vi "Configure Bus Source (Parallel).vi"(0 "VISA resource name":refnum<visa-resource-name>, 1 "Parallel Width (20)":dbl=20.0, 2 "Lock Clock":bool, 5 "BUS Number (9: Bus 1)":u16(ring)=9 items=["Bus 1"=9, "Bus 2"=10, "Bus 3"=11, "Bus 4"=12], 7 "Bit Source (0: Channel 1)":u16(ring) items=["Channel 1"=0, "Channel 2"=1, "Channel 3"=2, "Channel 4"=3, "Digital Channel 0"=14, "Digital Channel 1"=15, "Digital Channel 2"=16, "Digital Channel 3"=17, "Digital Channel 4"=18, "Digital Channel 5"=19, "Digital Channel 6"=20, "Digital Channel 7"=21, "Digital Channel 8"=22, "Digital Channel 9"=23, "Digital Channel 10"=24, "Digital Channel 11"=25, "Digital Channel 12"=26, "Digital Channel 13"=27, "Digital Channel 14"=28, "Digital Channel 15"=29], 9 "Clock Source (0: Channel 1)":u16(ring) items=["Channel 1"=0, "Channel 2"=1, "Channel 3"=2, "Channel 4"=3, "Digital Channel 0"=14, "Digital Channel 1"=15, "Digital Channel 2"=16, "Digital Channel 3"=17, "Digital Channel 4"=18, "Digital Channel 5"=19, "Digital Channel 6"=20, "Digital Channel 7"=21, "Digital Channel 8"=22, "Digital Channel 9"=23, "Digital Channel 10"=24, "Digital Channel 11"=25, "Digital Channel 12"=26, "Digital Channel 13"=27, "Digital Channel 14"=28, "Digital Channel 15"=29], 11 "error in (no error)":errorcluster, 12 "Bit Number (0: Normal)":u16(ring) items=["0", "1", "2", "3", "4", "5", "6", "7"], 13 "Clock Edge (0: Either)":u16(ring) items=["Either", "Rising", "Falling"]) -> (4 "VISA resource name out":refnum<visa-resource-name>, 15 "error out":errorcluster)   [LabVIEW 2010, in "Tektronix DPO MSO 2000 4000 Series.lvlib"]
doc: "This VI configures the Parallel bus.\n\n<B>Note:</B> This VI is only applicable for MSO3000 series."
uses:
  <instrlib>/Tektronix DPO MSO 2000 4000 Series/Tektronix DPO MSO 2000 4000 Series.lvlib
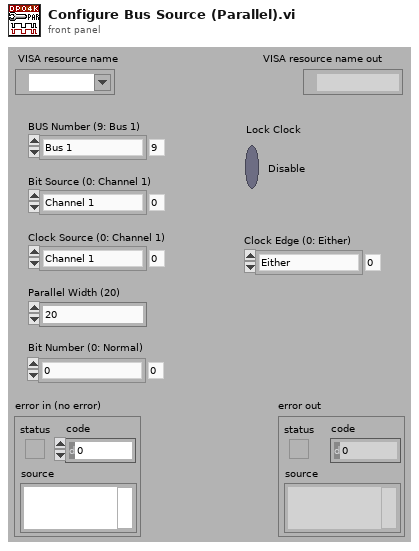
[diagram p1: front panel]
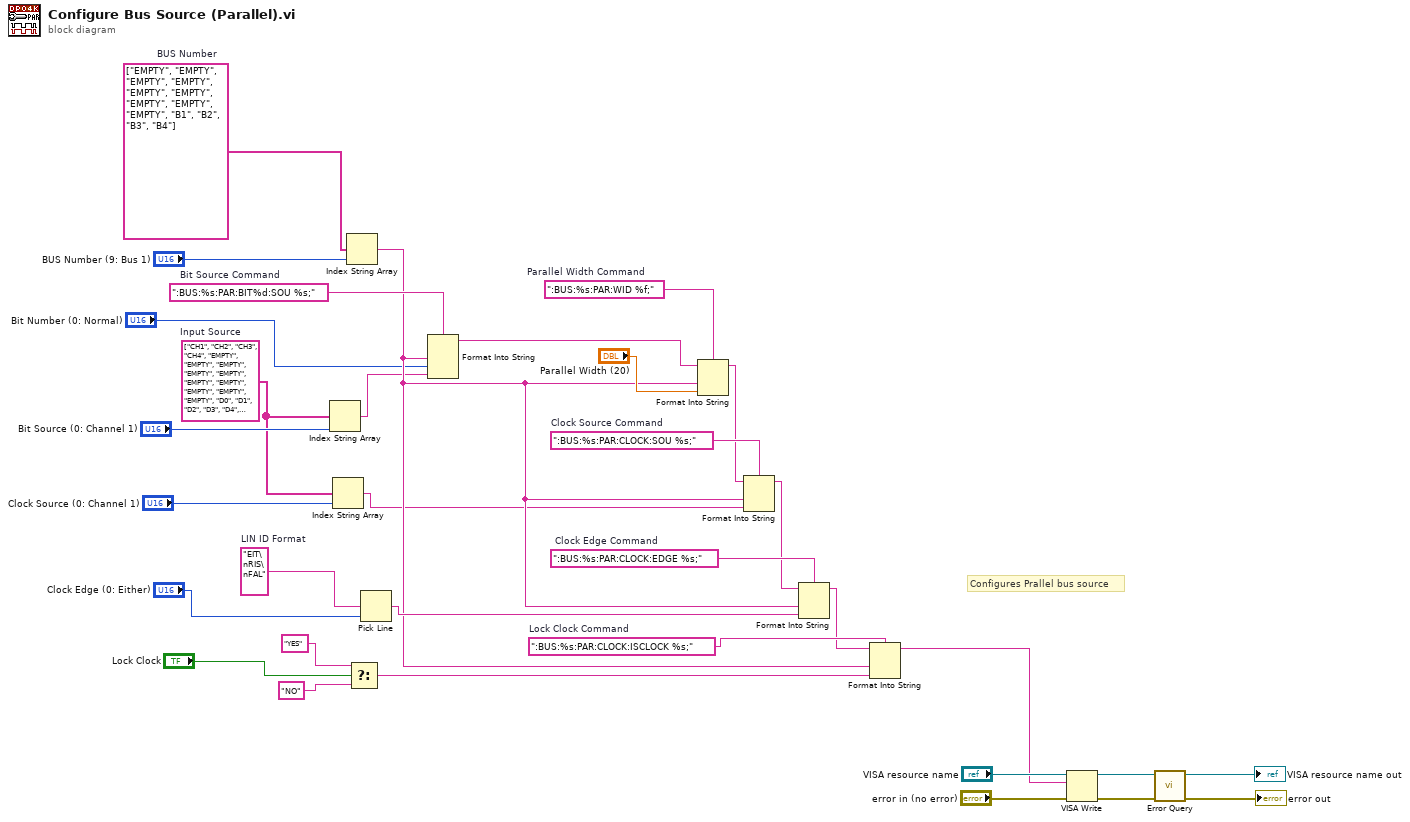
[diagram p0: block diagram]
diagram:
  w8 = string[] ["CH1", "CH2", "CH3", "CH4", "EMPTY", "EMPTY", "EMPTY", "EMPTY", "EMPTY", "EMPTY", "EMPTY", "EMPTY", "EMPTY", "EMPTY", "D0", "D1", "D2", "D3", "D4", "D5", "D6", "D7", "D8", "D9", "D10", "D11", "D12", "D13", "D14", "D15"]  # Input Source
  w13 = ":BUS:%s:PAR:CLOCK:ISCLOCK %s;"  # Lock Clock Command
  w17 = "EIT\nRIS\nFAL"  # LIN ID Format
  w19 = ":BUS:%s:PAR:CLOCK:EDGE %s;"  # Clock Edge Command
  w21 = ":BUS:%s:PAR:CLOCK:SOU %s;"  # Clock Source Command
  w23 = ":BUS:%s:PAR:WID %f;"  # Parallel Width Command
  w31 = ":BUS:%s:PAR:BIT%d:SOU %s;"  # Bit Source Command
  w32 = string[] ["EMPTY", "EMPTY", "EMPTY", "EMPTY", "EMPTY", "EMPTY", "EMPTY", "EMPTY", "EMPTY", "B1", "B2", "B3", "B4"]  # BUS Number
  # "Configures Prallel bus source"
  n1 = Index String Array(1:"Bit Source (0: Channel 1)", 2:w8) -> (0:w10:string)  [unwired: 1 in]
  n2 = Index String Array(1:"Clock Source (0: Channel 1)", 2:w8) -> (0:w6:string)  [unwired: 1 in]
  n3 = Index String Array(1:"BUS Number (9: Bus 1)", 2:w32) -> (0:w14:string)  [unwired: 1 in]
  n4 = Select(t="YES", s="Lock Clock", f="NO") -> (s? t:f=w2:string)
  n5 = Pick Line(multi-line string=w17, line index="Clock Edge (0: Either)") -> (output string=w15:string)  [unwired: 1 in]
  n6 = Format Into String(format string=w31, w14, "Bit Number (0: Normal)", w10) -> (resulting string=w30:string)  [unwired: 2 in, 1 out]
  n7 = Format Into String(format string=w23, initial string=w30, w14, "Parallel Width (20)") -> (resulting string=w20:string)  [unwired: 1 in, 1 out]
  n8 = Format Into String(format string=w21, initial string=w20, w14, w6) -> (resulting string=w18:string)  [unwired: 1 in, 1 out]
  n9 = Format Into String(format string=w19, initial string=w18, w14, w15) -> (resulting string=w12:string)  [unwired: 1 in, 1 out]
  n10 = Format Into String(format string=w13, initial string=w12, w14, w2) -> (resulting string=w1:string)  [unwired: 1 in, 1 out]
  n11 = VISA Write(VISA resource name="VISA resource name", write buffer=w1, error in (no error)="error in (no error)") -> (VISA resource name out=w27:refnum<visa-resource-name>, error out=w26:errorcluster)  [unwired: 1 out]
  n12 = call <instrlib>:"Error Query.vi"("error in (no error)"=w26, "VISA resource name"=w27) -> ("error out"=→"error out":errorcluster, "VISA resource name out"=→"VISA resource name out":refnum<visa-resource-name>)  [unwired: 6 in, 2 out]
